vi "libssh2_sftp_posix_rename_ex.vi"(8 "error in (no error)":errorcluster, 9 "destination file":string, 10 "source file":string, 11 "sftp":T1) -> (0 "error out":errorcluster)   [LabVIEW 2017, in "libssh2.lvlib"]
doc: "Rename a file or directory using POSIX semantics.\n\nPerforms a true rename operation, making it appear as if the file or directory has been moved to a new location.\n\n<B>Remarks</B>\nThis function is not supported by all SFTP servers."
uses:
  libssh2.lvlib
  SFTP Refnum.ctl
  Acquire Session.vi
  Release Session.vi
  Not An SFTP Refnum.vi
  <vilib>/Utility/error.llb/Error Cluster From Error Code.vi
  Global Settings.vi
  Read SFTP Refnum.vi
  Read Session Refnum.vi
  <vilib>/Utility/semaphor.llb/Acquire Semaphore.vi
  <vilib>/Utility/semaphor.llb/Release Semaphore.vi
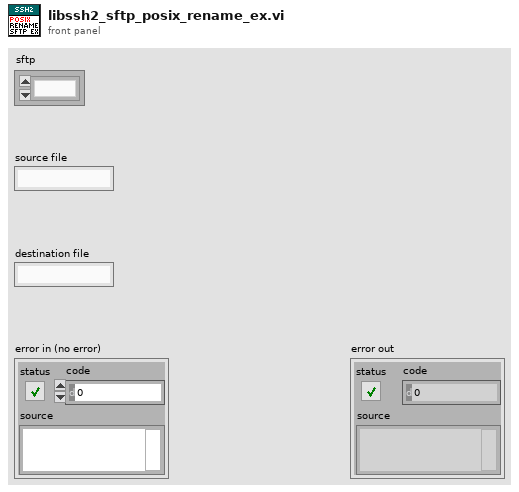
[diagram p1: front panel]
types:
  T1 = typedef "libssh2.lvlib/SFTP Refnum.ctl" = refnum<k1>
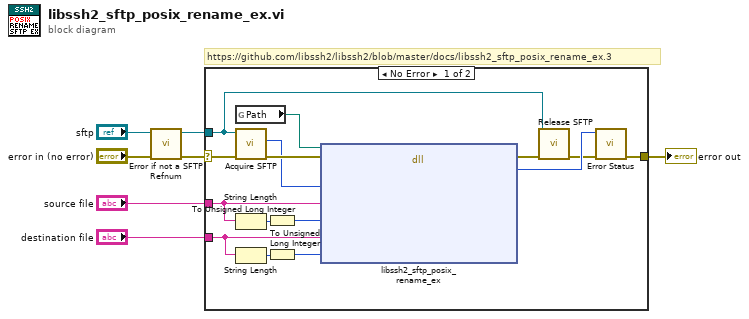
[diagram p0: block diagram]
diagram:
  # "https://github.com/libssh2/libssh2/blob/master/docs/libssh2_sftp_posix_rename_ex.3"
  n1 = call "Error if not a SFTP Refnum.vi"("error in (no error)"="error in (no error)", "sftp"="sftp") -> ("error out"=w6:errorcluster, "sftp out"=w5:T1)  [unwired: 8 in]
  n2 = case shown="No Error" w6 {
    selector: w6 -> [w21 w23]
    tunnel: w5 -> [w8 _]
    tunnel: [w17 w23] -> w4
    tunnel: "source file" -> [w15 _]
    tunnel: "destination file" -> [w10 _]
    frame No Error {
      n3 = global read "Global Settings.vi" "Path"() -> (w22:path)
      n4 = call "Acquire SFTP.vi"("error in (no error)"=w21, "sftp"=w8) -> ("error out"=w20:errorcluster, "LIBSSH2_SFTP*"=w19:u64)  [unwired: 8 in]
      n5 = String Length(string=w15) -> (length=w14:i32)
      n6 = String Length(string=w10) -> (length=w12:i32)
      n7 = To Unsigned Long Integer(number=w14) -> (unsigned 32bit integer=w13:u32)
      n8 = To Unsigned Long Integer(number=w12) -> (unsigned 32bit integer=w11:u32)
      n9 = dll-call lib="?" fn="libssh2_sftp_posix_rename_ex"(path in=w22, error in=w20, "sftp"=w19, "source_filename"=w15, "source_filename_len"=w13, "dest_filename"=w10, "dest_filename_len"=w11) -> (error out=w18:errorcluster, "return value"=w16:i32)  [unwired: 6 in, 1 out]
      n10 = call "Release SFTP.vi"("error in (no error)"=w18, "sftp"=w8) -> ("error out"=w9:errorcluster)  [unwired: 9 in]
      n11 = call "Error Status.vi"("error in (no error)"=w9, "return value"=w16) -> ("error out"=w17:errorcluster)  [unwired: 8 in, 1 out]
    }
    frame Error {
    }
  }
  "error out" <- w4
